vi "Get GRIP Data.vi"(8 "error in (no error)":errorcluster) -> (0 "error out":errorcluster, 2 "FPS":dbl, 3 "ContoursReport":T1[](array[typedef]))   [LabVIEW 2015]
uses:
  GRIP Contours Report.ctl
  <vilib>/Rock Robotics/Network Tables/NT Read Numeric Array.vi
  <vilib>/Rock Robotics/Network Tables/NT Read Number.vi
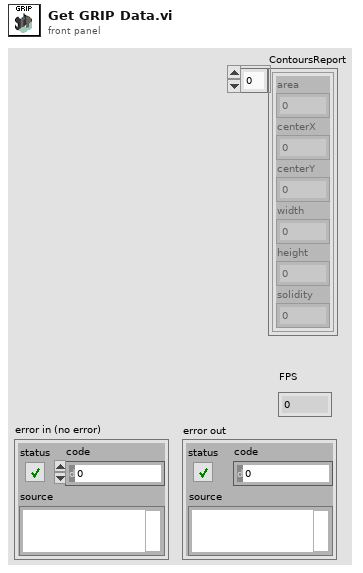
[diagram p1: front panel]
types:
  T1 = typedef "GRIP Contours Report.ctl" = cluster{"area":dbl, "centerX":dbl, "centerY":dbl, "width":dbl, "height":dbl, "solidity":dbl}
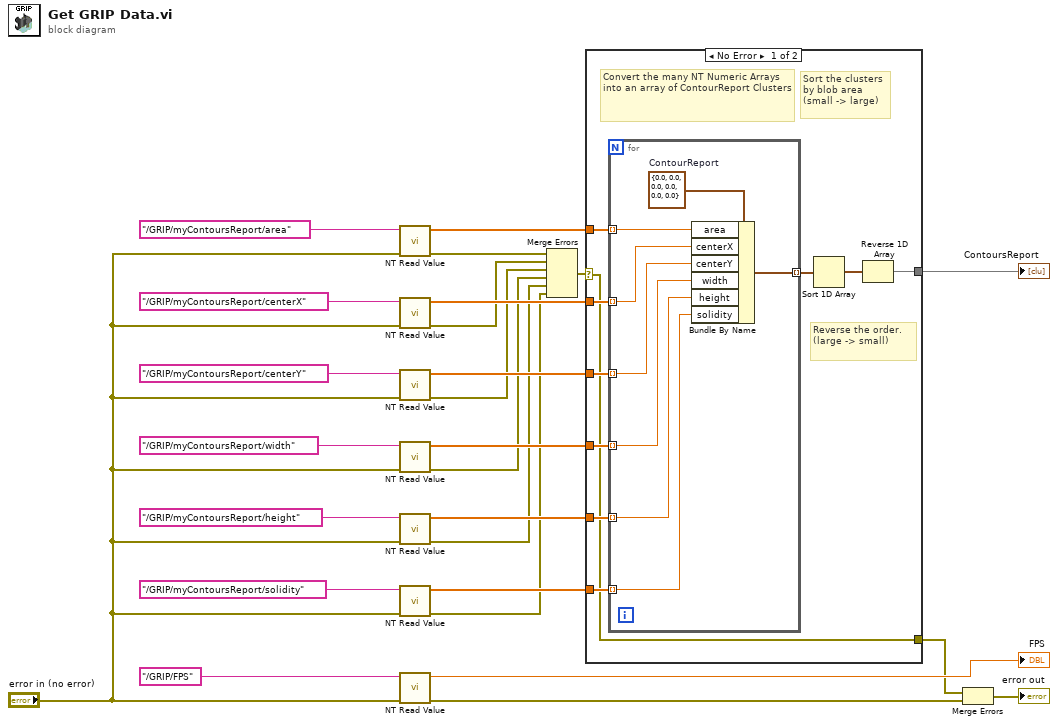
[diagram p0: block diagram]
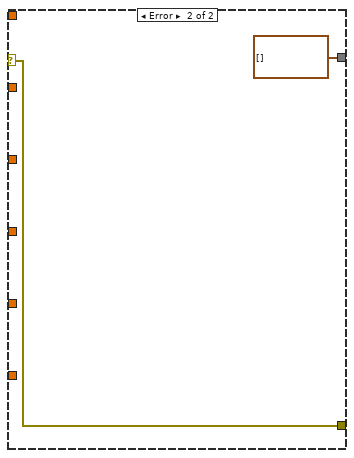
[diagram p2: hidden frame]
diagram:
  n1 = call-poly <vilib>:"NT Read Value.vi"("error in"="error in (no error)", "Name"="/GRIP/myContoursReport/area") -> ("error out"=w11:errorcluster, "Numeric Array"=w13:dbl[])  [unwired: 8 in]
  n2 = call-poly <vilib>:"NT Read Value.vi"("error in"="error in (no error)", "Name"="/GRIP/myContoursReport/centerX") -> ("error out"=w6:errorcluster, "Numeric Array"=w14:dbl[])  [unwired: 8 in]
  n3 = call-poly <vilib>:"NT Read Value.vi"("error in"="error in (no error)", "Name"="/GRIP/myContoursReport/centerY") -> ("error out"=w7:errorcluster, "Numeric Array"=w15:dbl[])  [unwired: 8 in]
  n4 = call-poly <vilib>:"NT Read Value.vi"("error in"="error in (no error)", "Name"="/GRIP/myContoursReport/width") -> ("error out"=w8:errorcluster, "Numeric Array"=w16:dbl[])  [unwired: 8 in]
  n5 = call-poly <vilib>:"NT Read Value.vi"("error in"="error in (no error)", "Name"="/GRIP/myContoursReport/height") -> ("error out"=w9:errorcluster, "Numeric Array"=w17:dbl[])  [unwired: 8 in]
  n6 = call-poly <vilib>:"NT Read Value.vi"("error in"="error in (no error)", "Name"="/GRIP/myContoursReport/solidity") -> ("error out"=w10:errorcluster, "Numeric Array"=w18:dbl[])  [unwired: 8 in]
  n7 = call-poly <vilib>:"NT Read Value.vi"("error in"="error in (no error)", "Name"="/GRIP/FPS" ("Variable")) -> ("error out"=w3:errorcluster, "Numeric"=→"FPS":dbl)  [unwired: 8 in]
  n8 = Merge Errors(w11, w6, w7, w8, w9, w10) -> (w5:errorcluster)
  n9 = case shown="No Error" w5 {
    selector: w5 -> [w27 w45]
    tunnel: w18 -> [w36 _]
    tunnel: w17 -> [w35 _]
    tunnel: w16 -> [w34 _]
    tunnel: w15 -> [w33 _]
    tunnel: w14 -> [w32 _]
    tunnel: w13 -> [w31 _]
    tunnel: [w28 T1[] []] -> w12
    tunnel: [w27 w45] -> w4
    frame No Error {
      # "Reverse the order.\n(large -> small)"
      # "Sort the clusters by blob area\n(small -> large)"
      # "Convert the many NT Numeric Arrays into an array of ContourReport Clusters"
      n10 = for {
        tunnel: w36 -> [w42] mode=indexing
        tunnel: w35 -> [w41] mode=indexing
        tunnel: w34 -> [w40] mode=indexing
        tunnel: w33 -> [w39] mode=indexing
        tunnel: w32 -> [w38] mode=indexing
        tunnel: w31 -> [w43] mode=indexing
        tunnel: [w37] -> w30 mode=indexing
        w44 = T1 {"area"=0.0, "centerX"=0.0, "centerY"=0.0, "width"=0.0, "height"=0.0, "solidity"=0.0}  # ContourReport
        n11 = Bundle By Name(cluster=w44, "area"=w43, "centerX"=w38, "centerY"=w39, "width"=w40, "height"=w41, "solidity"=w42) -> (w37:T1)
      }
      n12 = Sort 1D Array(array=w30) -> (sorted array=w29:T1[])
      n13 = Reverse 1D Array(array=w29) -> (reversed array=w28:T1[])
    }
    frame Error {
    }
  }
  "ContoursReport" <- w12
  n14 = Merge Errors(w4, w3) -> (→"error out":errorcluster)
